vi "VI_Sort2DArray.vi"(8 "error in (no error)":errorcluster, 10 "Collumn to sort by":i16, 11 "Array In":string[][](array[string])) -> (0 "error out":errorcluster, 3 "Array Out":string[][](array[string]))   [LabVIEW 2018]
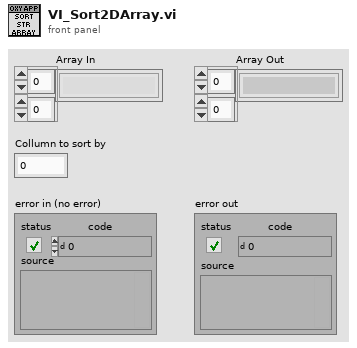
[diagram p1: front panel]
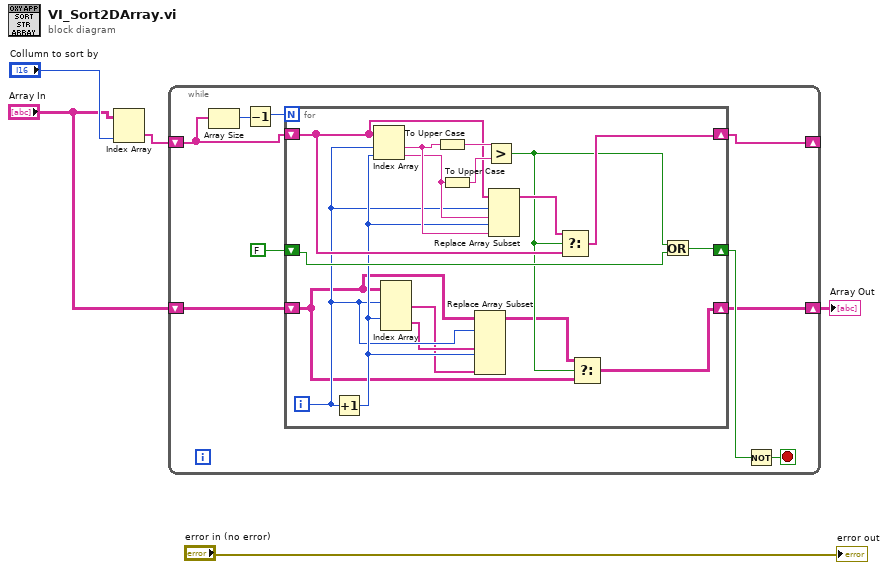
[diagram p0: block diagram]
diagram:
  n1 = Index Array(array="Array In", index (col)="Collumn to sort by") -> (element=w4:string[])  [unwired: 1 in]
  n2 = while {
    shift-right: [w10] -> _
    shift-left: w4 -> [w11]
    shift-right: [w6] -> w2
    shift-left: "Array In" -> [w7]
    stop <- w8 stop-if-true
    n3 = Array Size(array=w11) -> (size(s)=w13:i32)
    n4 = Decrement(x=w13) -> (x-1=w12:i32)
    n5 = for {
      N: w12 -> [_]
      shift-right: [w28] -> w9
      shift-left: FALSE -> [w29]
      shift-right: [w24] -> w10
      shift-left: w11 -> [w27]
      shift-right: [w21] -> w6
      shift-left: w7 -> [w17]
      i -> [w18]
      n6 = Increment(x=w18) -> (x+1=w19:i32)
      n7 = Index Array(array=w27, index #1=w18, index #2=w19) -> (element #1=w26:string, element #2=w20:string)
      n8 = Index Array(array=w17, index (row) #1=w18, index (row) #2=w19) -> (element #1=w15:string[], element #2=w16:string[])  [unwired: 2 in]
      n9 = To Upper Case(1:w26) -> (0:w31:string)
      n10 = To Upper Case(1:w20) -> (0:w30:string)
      n11 = Replace Array Subset(array=w17, new element #1=w16, index (row) #1=w18, new element #2=w15, index (row) #2=w19) -> (w22:string[][])  [unwired: 2 in]
      n12 = Greater?(x=w31, y=w30) -> (0:w23:bool)
      n13 = Replace Array Subset(array=w27, new element #1=w20, index #1=w18, new element #2=w26, index #2=w19) -> (w25:string[])
      n14 = Select(t=w25, s=w23, f=w27) -> (s? t:f=w24:string[])
      n15 = Select(t=w22, s=w23, f=w17) -> (s? t:f=w21:string[][])
      n16 = Or(x=w23, y=w29) -> (x .or. y?=w28:bool)
    }
    n17 = Not(x=w9) -> (.not. x?=w8:bool)
  }
  "Array Out" <- w2
  "error out" <- "error in (no error)"
